vi "Refresh Statistics.vi"(11 "CIFPlugin in":refnum<class "Template_Plugin.lvclass">) -> (3 "CIFPlugin out":refnum<class "Template_Plugin.lvclass">)   [LabVIEW 2021, in "Template_Plugin.lvclass"]
uses:
  Template_Plugin.lvclass
  Template_Plugin.lvclass/Template_Plugin.ctl
  Typedef/Statistics.ctl
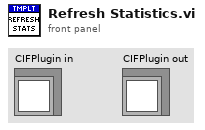
[diagram p1: front panel]
types:
  T1 = typedef "Template_Plugin.lvclass/Statistics.ctl" = cluster{"Iterations":u64}
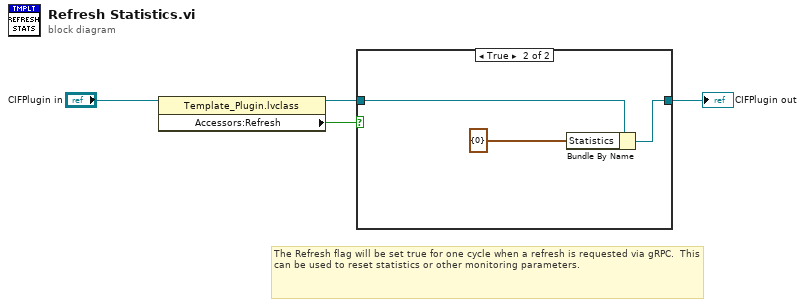
[diagram p0: block diagram]
diagram:
  # "The Refresh flag will be set true for one cycle when a refresh is requested via gRPC.  This can be used to reset statistics or other monitoring parameters."
  n1 = property class="Template_Plugin.lvclass"(reference="CIFPlugin in") -> (reference out=w2:refnum<class "Template_Plugin.lvclass">, "Accessors:Refresh"=w3:bool)  [unwired: 1 in, 1 out]
  n2 = case shown="True" w3 {
    tunnel: w2 -> [w5 w8]
    tunnel: [w5 w7] -> w1
    frame False {
    }
    frame True {
      n3 = Bundle By Name(cluster=w8, "Statistics"=T1 {"Iterations"=0} ("-> gRPC Comm.Cyclic Data -> gRPC .Statistics")) -> (w7:refnum<class "Template_Plugin.lvclass">)
    }
  }
  "CIFPlugin out" <- w1
